vi "Write ID.vi"(8 "error in (no error)":errorcluster, 10 "ID":string, 11 "Update Data MSG in":refnum<class "Update Data MSG.lvclass">) -> (0 "error out":errorcluster, 3 "Update Data MSG out":refnum<class "Update Data MSG.lvclass">)   [LabVIEW 2014, in "Controller.lvlib" / "Update Data MSG.lvclass"]
uses:
  Update Data MSG.lvclass
  Update Data MSG.lvclass/Update Data MSG.ctl
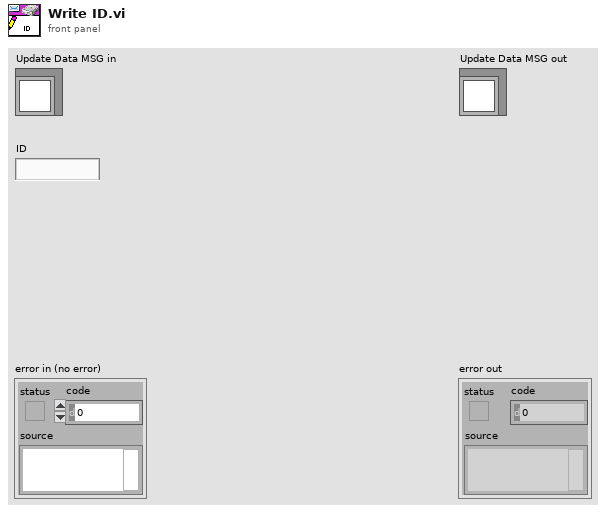
[diagram p1: front panel]
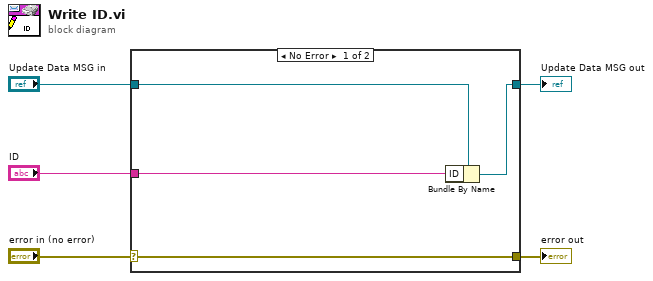
[diagram p0: block diagram]
diagram:
  n1 = case shown="No Error" "error in (no error)" {
    selector: "error in (no error)" -> [w9 w10]
    tunnel: [w9 w10] -> w4
    tunnel: [w7 w11] -> w2
    tunnel: "Update Data MSG in" -> [w8 w11]
    tunnel: "ID" -> [w6 _]
    frame No Error {
      n2 = Bundle By Name(cluster=w8, "ID"=w6) -> (w7:refnum<class "Update Data MSG.lvclass">)
    }
    frame Error {
    }
  }
  "error out" <- w4
  "Update Data MSG out" <- w2
